vi "主程序.vi"() -> ()   [LabVIEW 2010]
panel:
  out "number：0 to 1":dbl
  out "loop number":dbl
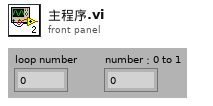
[diagram p1: front panel]
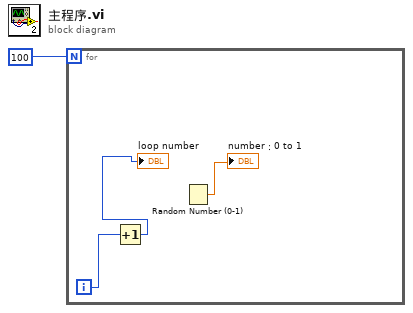
[diagram p0: block diagram]
diagram:
  n1 = for {
    N: 100 -> [_]
    i -> [w4]
    n2 = Increment(x=w4) -> (x+1=→"loop number":i32)
    n3 = Random Number (0-1)() -> (number: 0 to 1=→"number：0 to 1":dbl)
  }
